vi "Fields to Detailed Fields.vi"(10 "Fields":string[](array[string]), 11 "Table Name":string) -> (3 "Detailed Fields":string[](array[string]))   [LabVIEW 2021, in "EDT SQLite+.lvlib"]
uses:
  EDT SQLite+.lvlib
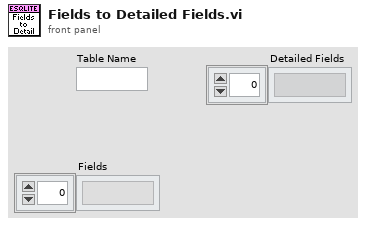
[diagram p1: front panel]
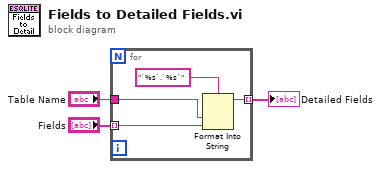
[diagram p0: block diagram]
diagram:
  n1 = for {
    tunnel: "Fields" -> [w7] mode=indexing
    tunnel: [w5] -> w1 mode=indexing
    tunnel: "Table Name" -> [w4]
    n2 = Format Into String(format string="`%s`.`%s`", w4, w7) -> (resulting string=w5:string)  [unwired: 2 in, 1 out]
  }
  "Detailed Fields" <- w1
